vi "SVT UFF58 Open File.vi"(0 "UFF58 file path":path, 5 "open mode (create:0)":T2, 9 "byte order (2:little-endian)":T1(ring)=enum."little-endian", 11 "error in (no error)":errorcluster) -> (4 "file refnum":refnum<k20>, 6 "UFF58 file path out":path, 15 "error out":errorcluster)   [LabVIEW 2017, in "SoundVib_UFF58.lvlib"]
doc: "Opens an existing UFF58 (universal file format) file, creates a new UFF58 file, or replaces an existing UFF file. You can input the file programmatically or interactively using a file dialog box."
uses:
  <vilib>/addons/Sound and Vibration/svt_UFF58/SoundVib_UFF58.lvlib
  <vilib>/addons/Sound and Vibration/svt_UFF58/subVIs/sv_UFF58 Open Mode.ctl
  <vilib>/Platform/storage/lvStorage.llb/_openFunction.ctl
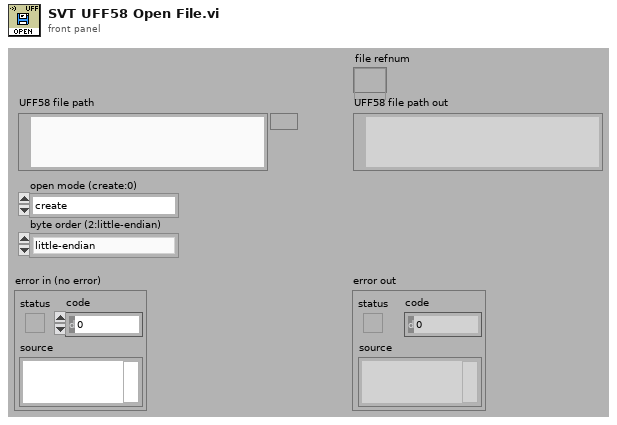
[diagram p1: front panel]
types:
  T1 = enum16{"big-endian, network order", "native, host order", "little-endian"}
  T2 = typedef "SoundVib_UFF58.lvlib/sv_UFF58 Open Mode.ctl" = enum16{"create ", "create or replace", "open (read only)"}
  T3 = typedef "_openFunction.ctl" = enum16{"open", "open or create", "create or replace", "create", "open (read only)"}
  T4 = enum32{"existing file", "new file", "new or existing file", "existing dir", "new dir", "new or existing dir", "existing file (use LLBs)", "new file (use LLBs)", "new or existing file (use LLBs)", "new or existing file or directory (use LLBs)"}
  T5 = enum16{"existing file", "new file", "new or existing file", "existing dir", "new dir", "new or existing dir"}[]
  T6 = enum16{"existing file", "new file", "new or existing file", "existing dir", "new dir", "new or existing dir"}
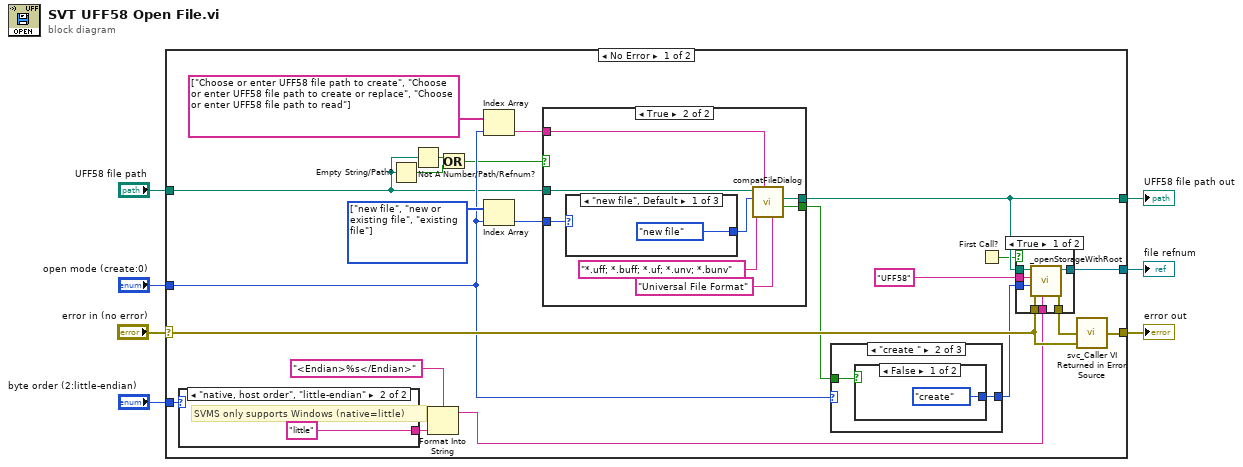
[diagram p0: block diagram]
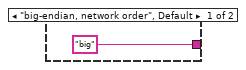
[diagram p2: hidden frame]
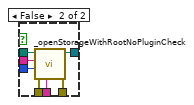
[diagram p3: hidden frame]
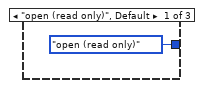
[diagram p4: hidden frame]
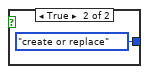
[diagram p5: hidden frame]
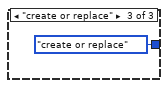
[diagram p6: hidden frame]
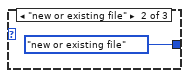
[diagram p8: hidden frame]
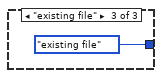
[diagram p9: hidden frame]
diagram:
  n1 = case shown="No Error" "error in (no error)" {
    selector: "error in (no error)" -> [w27 w65]
    tunnel: "UFF58 file path" -> [w14 w64]
    tunnel: "open mode (create:0)" -> [w19 _]
    tunnel: [w26 w65] -> w6
    tunnel: [w29 _] -> w5
    tunnel: [w17 w64] -> w2
    tunnel: "byte order (2:little-endian)" -> [w11 _]
    frame No Error {
      w23 = T5 [enum."new file", enum."new or existing file", enum."existing file"] items=["existing file", "new file", "new or existing file", "existing dir", "new dir", "new or existing dir"]
      n2 = case shown="\"native, host order\", \"little-endian\"" w11 {
        tunnel: ["big" ("pattern label") "little" ("pattern label")] -> w9
        frame "big-endian, network order", Default {
        }
        frame "native, host order", "little-endian" {
          # "SVMS only supports Windows (native=little)"
        }
      }
      n3 = Empty String/Path?(string/path=w14) -> (empty?=w15:bool)
      n4 = Not A Number/Path/Refnum?(number/path/refnum=w14) -> (NaN/Path/Refnum?=w16:bool)
      n5 = Format Into String(format string="<Endian>%s</Endian>" ("pattern label"), w9) -> (resulting string=w8:string)  [unwired: 2 in, 1 out]
      n6 = Or(x=w16, y=w15) -> (x .or. y?=w13:bool)
      n7 = Index Array(array=string[] ["Choose or enter UFF58 file path to create", "Choose or enter UFF58 file path to create or replace", "Choose or enter UFF58 file path to read"], index=w19) -> (element=w18:string)
      n8 = Index Array(array=w23, index=w19) -> (element=w22:T6)
      n9 = case shown="True" w13 {
        tunnel: w14 -> [w52 w58]
        tunnel: [w52 w57] -> w17
        tunnel: w22 -> [_ w54]
        tunnel: [_ w56] -> w21
        tunnel: w18 -> [_ w55]
        frame False {
        }
        frame True {
          n10 = case shown="\"new file\", Default" w54 {
            tunnel: [T4."new file" ("select mode (2)") T4."new or existing file" ("select mode (2)") T4."existing file" ("select mode (2)")] -> w53
            frame "new file", Default {
            }
            frame "new or existing file" {
            }
            frame "existing file" {
            }
          }
          n11 = call <vilib>:"compatFileDialog.vi"("pattern label"="Universal File Format", "prompt"=w55, "pattern"="*.uff; *.buff; *.uf; *.unv; *.bunv", "select mode (2)"=w53, "start path"=w58) -> ("exists"=w56:bool, "path"=w57:path)  [unwired: 4 in, 1 out]
        }
      }
      n12 = case shown="\"create \"" w19 {
        tunnel: [_openFunction."open (read only)" ("open mode (open:0)") w48 _openFunction."create or replace" ("open mode (open:0)")] -> w24
        tunnel: w21 -> [_ w47 _]
        frame "open (read only)", Default {
        }
        frame "create " {
          n13 = case shown="False" w47 {
            tunnel: [_openFunction."create" ("open mode (open:0)") _openFunction."create or replace" ("open mode (open:0)")] -> w48
            frame False {
            }
            frame True {
            }
          }
        }
        frame "create or replace" {
        }
      }
      n14 = First Call?() -> (First Call?: T/F=w12:bool)
      n15 = case shown="True" w12 {
        tunnel: [w38 w45] -> w29
        tunnel: [w37 w44] -> w28
        tunnel: w27 -> [w36 w43]
        tunnel: "UFF58" ("Storage Format") -> [w35 w42]
        tunnel: w24 -> [w34 w41]
        tunnel: w17 -> [w33 w40]
        tunnel: w8 -> [w32 w39]
        frame True {
          n16 = call <vilib>:"_openStorageWithRoot.vi"("Additional parameters"=w32, "error in (no error)"=w36, "Overwrite Options"=w34, "Storage Format"=w35, "Storage Location"=w33) -> ("error out"=w37:errorcluster, "Data Object"=w38:refnum<k20>)  [unwired: 5 in]
        }
        frame False {
          n17 = call <vilib>:"_openStorageWithRootNoPluginCheck.vi"("Additional parameters"=w39, "error in (no error)"=w43, "Overwrite Options"=w41, "Storage Format"=w42, "Storage Location"=w40) -> ("error out"=w44:errorcluster, "Data Object"=w45:refnum<k20>)  [unwired: 5 in]
        }
      }
      n18 = call <vilib>:"svc_Caller VI Returned in Error Source.vi"("warning input to caller"=w27, "error in (no error)"=w28) -> ("error out"=w26:errorcluster)  [unwired: 3 in]
    }
    frame Error {
    }
  }
  "error out" <- w6
  "file refnum" <- w5
  "UFF58 file path out" <- w2
